vi "tm3samp_10_dualsync.vi"() -> ()   [LabVIEW 2011]
panel:
  out "Camera Model":string
  out "Image":u16[][](graph)
  in  "capture":bool
  in  "Quit":bool
  out "Error Out":errorcluster {"code" format="%.0x"}
  # "This is an example of one way\nto synchronize two of the same\nmodel cameras."
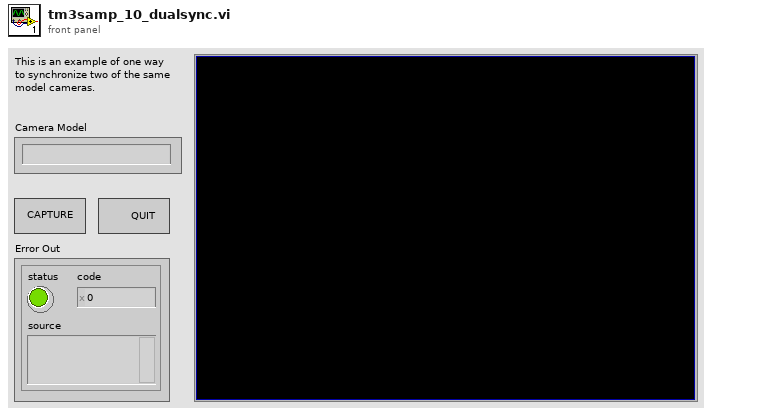
[diagram p1: front panel]
types:
  T1 = cluster{"height":u32, "width":u32, "datatype":u32}
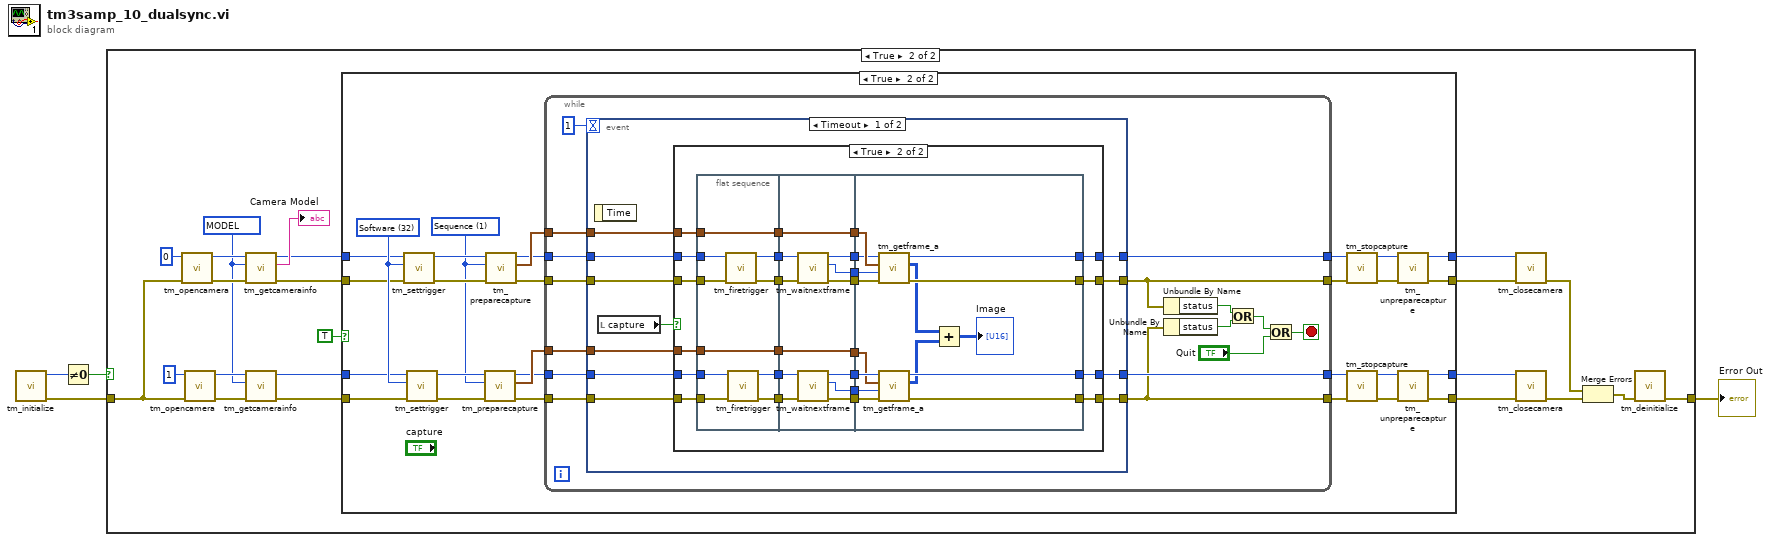
[diagram p0: block diagram]
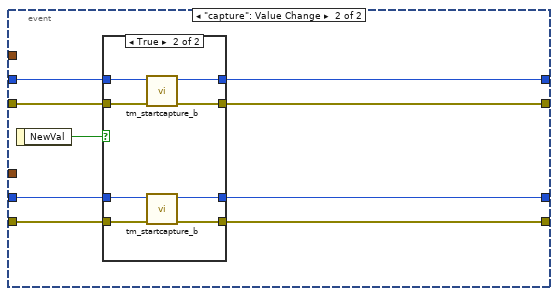
[diagram p5: hidden frame]
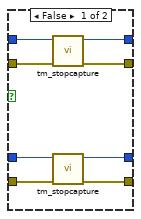
[diagram p6: hidden frame]
diagram:
  n1 = call <userlib>:"tm_initialize.vi"() -> ("error out"=w1:errorcluster, "Number Of Cameras"=w2:u32)  [unwired: 8 in, 2 out]
  n2 = Not Equal To 0?(x=w2) -> (x != 0?=w4:bool)
  n3 = case shown="True" w4 {
    tunnel: w1 -> [w5 w24]
    tunnel: [w5 w26] -> w3
    frame False {
    }
    frame True {
      w16 = u32 67109124 items=["BUS"=67109121, "CAMERA ID"=67109122, "VENDOR"=67109123, "MODEL"=67109124, "CAMERA VERSION"=67109125, "DRIVER VERSION"=67109126, "MODULE VERSIOIN"=67109127, "DCAMAPI VERSION"=67109128] ("Info ID")
      n4 = call <userlib>:"tm_opencamera.vi"("error in (no error)"=w24, "Camera Index"=u32 0) -> ("error out"=w19:errorcluster, "Handle out"=w20:u32)  [unwired: 7 in, 1 out]
      n5 = call <userlib>:"tm_opencamera.vi"("error in (no error)"=w24, "Camera Index"=u32 1) -> ("error out"=w17:errorcluster, "Handle out"=w18:u32)  [unwired: 7 in, 1 out]
      n6 = call <userlib>:"tm_getcamerainfo.vi"("error in (no error)"=w19, "Info ID"=w16, "Handle in"=w20) -> ("error out"=w12:errorcluster, "String"=→"Camera Model":string, "Handle out"=w11:u32)  [unwired: 6 in]
      n7 = call <userlib>:"tm_getcamerainfo.vi"("error in (no error)"=w17, "Info ID"=w16, "Handle in"=w18) -> ("error out"=w13:errorcluster, "Handle out"=w14:u32)  [unwired: 6 in, 1 out]
      n8 = case shown="True" TRUE {
        tunnel: w14 -> [w31 w41]
        tunnel: w13 -> [w30 w40]
        tunnel: w12 -> [w29 w36]
        tunnel: w11 -> [w28 w37]
        tunnel: [w31 w43] -> w10
        tunnel: [w30 w42] -> w9
        tunnel: [w29 w38] -> w8
        tunnel: [w28 w39] -> w7
        frame False {
        }
        frame True {
          w44 = u32 32 items=["Internal"=1, "External Edge"=2, "External Level"=4, "Software"=32, "Fast Repetition"=64, "TDI"=128, "Trigger Start"=512, "Sync Readout"=1024] ("Trigger Mode")
          w45 = 1 items=["Snap", "Sequence"] ("Capture mode")
          n9 = call <userlib>:"tm_settrigger.vi"("error in (no error)"=w36, "Trigger Mode"=w44, "Handle in"=w37) -> ("error out"=w51:errorcluster, "Handle out"=w52:u32)  [unwired: 7 in]
          n10 = call <userlib>:"tm_settrigger.vi"("error in (no error)"=w40, "Trigger Mode"=w44, "Handle in"=w41) -> ("error out"=w53:errorcluster, "Handle out"=w54:u32)  [unwired: 7 in]
          n11 = call <userlib>:"tm_preparecapture.vi"("error in (no error)"=w53, "Capture mode"=w45, "Handle in"=w54) -> ("error out"=w32:errorcluster, "Buffer Info"=w59:T1, "Handle out"=w33:u32)  [unwired: 5 in, 1 out]
          n12 = call <userlib>:"tm_preparecapture.vi"("error in (no error)"=w51, "Capture mode"=w45, "Handle in"=w52) -> ("error out"=w35:errorcluster, "Buffer Info"=w50:T1, "Handle out"=w34:u32)  [unwired: 5 in, 1 out]
          n13 = while {
            tunnel: [w73] -> w58
            tunnel: [w65] -> w57
            tunnel: w33 -> [w75]
            tunnel: w32 -> [w74]
            tunnel: w59 -> [w72]
            tunnel: w34 -> [w69]
            tunnel: w35 -> [w68]
            tunnel: w50 -> [w67]
            tunnel: [w64] -> w46
            tunnel: [w66] -> w47
            stop <- w62 stop-if-true
            n14 = event shown="[0] Timeout" {
              selector: _ -> [_ _]
              dyn-events: _ -> [_ _]
              timeout: 1 -> [_ _]
              tunnel: w75 -> [w81 w159]
              tunnel: w74 -> [w80 w158]
              tunnel: [w77 w157] -> w73
              tunnel: [w76 w156] -> w65
              tunnel: w72 -> [w82 _]
              tunnel: w69 -> [w84 w155]
              tunnel: w67 -> [w85 _]
              tunnel: w68 -> [w83 w154]
              tunnel: [w78 w152] -> w66
              tunnel: [w79 w153] -> w64
              event Timeout {
                n15 = event-data() -> ()  [unwired: 1 in, 1 out]
                n16 = local read "capture"() -> (w86:bool)
                n17 = case shown="True" w86 {
                  tunnel: w85 -> [_ w102]
                  tunnel: w84 -> [w90 w101]
                  tunnel: w83 -> [w89 w100]
                  tunnel: w82 -> [_ w99]
                  tunnel: w81 -> [w87 w98]
                  tunnel: w80 -> [w88 w97]
                  tunnel: [w89 w96] -> w79
                  tunnel: [w90 w95] -> w78
                  tunnel: [w87 w94] -> w77
                  tunnel: [w88 w93] -> w76
                  frame False {
                  }
                  frame True {
                    n18 = flat-sequence {
                      tunnel: w98 -> [w124]
                      tunnel: w97 -> [w123]
                      tunnel: [w122] -> w114
                      tunnel: [w121] -> w113
                      tunnel: w99 -> [w120]
                      tunnel: [w120] -> w112
                      tunnel: w102 -> [w119]
                      tunnel: [w119] -> w111
                      tunnel: w101 -> [w118]
                      tunnel: [w116] -> w110
                      tunnel: w100 -> [w117]
                      tunnel: [w115] -> w109
                      tunnel: w114 -> [w133]
                      tunnel: w113 -> [w134]
                      tunnel: w112 -> [w127]
                      tunnel: w111 -> [w132]
                      tunnel: w110 -> [w135]
                      tunnel: w109 -> [w136]
                      tunnel: [w132] -> w108
                      tunnel: [w131] -> w107
                      tunnel: [w130] -> w106
                      tunnel: [w129] -> w105
                      tunnel: [w128] -> w104
                      tunnel: [w127] -> w103
                      tunnel: [w125] -> w92
                      tunnel: [w126] -> w91
                      tunnel: w108 -> [w151]
                      tunnel: w107 -> [w149]
                      tunnel: w106 -> [w150]
                      tunnel: [w148] -> w95
                      tunnel: [w147] -> w96
                      tunnel: w105 -> [w146]
                      tunnel: w104 -> [w145]
                      tunnel: w103 -> [w144]
                      tunnel: [w143] -> w94
                      tunnel: [w142] -> w93
                      tunnel: w92 -> [w141]
                      tunnel: w91 -> [w140]
                      frame #0 {
                        n19 = call <userlib>:"tm_firetrigger.vi"("error in (no error)"=w117, "Handle in"=w118) -> ("error out"=w115:errorcluster, "Handle out"=w116:u32)  [unwired: 8 in]
                        n20 = call <userlib>:"tm_firetrigger.vi"("error in (no error)"=w123, "Handle in"=w124) -> ("error out"=w121:errorcluster, "Handle out"=w122:u32)  [unwired: 8 in]
                      }
                      frame #1 {
                        n21 = call <userlib>:"tm_waitnextframe.vi"("error in (no error)"=w136, "Handle in"=w135) -> ("error out"=w130:errorcluster, "Frame Index"=w125:i32, "Handle out"=w131:u32)  [unwired: 6 in, 1 out]
                        n22 = call <userlib>:"tm_waitnextframe.vi"("error in (no error)"=w134, "Handle in"=w133) -> ("error out"=w128:errorcluster, "Frame Index"=w126:i32, "Handle out"=w129:u32)  [unwired: 6 in, 1 out]
                      }
                      frame #2 {
                        n23 = call <userlib>:"tm_getframe_a.vi"("error in (no error)"=w150, "Frame Index"=w141, "Buffer Info"=w151, "Handle in"=w149) -> ("error out"=w147:errorcluster, "Data 16"=w139:u16[][], "Handle out"=w148:u32)  [unwired: 3 in, 2 out]
                        n24 = call <userlib>:"tm_getframe_a.vi"("error in (no error)"=w145, "Frame Index"=w140, "Buffer Info"=w144, "Handle in"=w146) -> ("error out"=w142:errorcluster, "Data 16"=w138:u16[][], "Handle out"=w143:u32)  [unwired: 3 in, 2 out]
                        n25 = Add(x=w139, y=w138) -> (x+y=→"Image":u16[][])
                      }
                    }
                  }
                }
              }
              event "capture": Value Change {
                n26 = event-data() -> ("NewVal"=w160:bool)  [unwired: 1 in]
                n27 = case shown="True" w160 {
                  tunnel: w159 -> [w168 w176]
                  tunnel: w158 -> [w167 w175]
                  tunnel: [w166 w174] -> w157
                  tunnel: [w165 w173] -> w156
                  tunnel: w155 -> [w163 w172]
                  tunnel: w154 -> [w164 w171]
                  tunnel: [w162 w170] -> w152
                  tunnel: [w161 w169] -> w153
                  frame False {
                    n28 = call <userlib>:"tm_stopcapture.vi"("error in (no error)"=w164, "Handle in"=w163) -> ("error out"=w161:errorcluster, "Handle out"=w162:u32)  [unwired: 8 in]
                    n29 = call <userlib>:"tm_stopcapture.vi"("error in (no error)"=w167, "Handle in"=w168) -> ("error out"=w165:errorcluster, "Handle out"=w166:u32)  [unwired: 8 in]
                  }
                  frame True {
                    n30 = call <userlib>:"tm_startcapture_b.vi"("error in (no error)"=w171, "Handle in"=w172) -> ("error out"=w169:errorcluster, "Handle out"=w170:u32)  [unwired: 8 in]
                    n31 = call <userlib>:"tm_startcapture_b.vi"("error in (no error)"=w175, "Handle in"=w176) -> ("error out"=w173:errorcluster, "Handle out"=w174:u32)  [unwired: 8 in]
                  }
                }
              }
            }
            n32 = Unbundle By Name(w64) -> ("status"=w71:bool)
            n33 = Unbundle By Name(w65) -> ("status"=w63:bool)
            n34 = Or(x=w71, y=w63) -> (x .or. y?=w61:bool)
            n35 = Or(x=w61, y="Quit") -> (x .or. y?=w62:bool)
          }
          n36 = call <userlib>:"tm_stopcapture.vi"("error in (no error)"=w46, "Handle in"=w47) -> ("error out"=w48:errorcluster, "Handle out"=w49:u32)  [unwired: 8 in]
          n37 = call <userlib>:"tm_stopcapture.vi"("error in (no error)"=w57, "Handle in"=w58) -> ("error out"=w55:errorcluster, "Handle out"=w56:u32)  [unwired: 8 in]
          n38 = call <userlib>:"tm_unpreparecapture.vi"("error in (no error)"=w48, "Handle in"=w49) -> ("error out"=w38:errorcluster, "Handle out"=w39:u32)  [unwired: 8 in]
          n39 = call <userlib>:"tm_unpreparecapture.vi"("error in (no error)"=w55, "Handle in"=w56) -> ("error out"=w42:errorcluster, "Handle out"=w43:u32)  [unwired: 8 in]
        }
      }
      n40 = call <userlib>:"tm_closecamera.vi"("error in (no error)"=w8, "Handle in"=w7) -> ("error out"=w23:errorcluster)  [unwired: 9 in]
      n41 = call <userlib>:"tm_closecamera.vi"("error in (no error)"=w9, "Handle in"=w10) -> ("error out"=w22:errorcluster)  [unwired: 9 in]
      n42 = Merge Errors(w23, w22) -> (w21:errorcluster)
      n43 = call <userlib>:"tm_deinitialize.vi"("error in (no error)"=w21) -> ("error out"=w26:errorcluster)  [unwired: 10 in]
    }
  }
  "Error Out" <- w3
